vi "indexed_analog.vi"() -> ()   [LabVIEW 2018]
panel:
  in  "Index":u16
  in  "Analog":fxp<+/-,24,5>
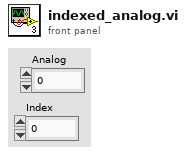
[diagram p1: front panel]
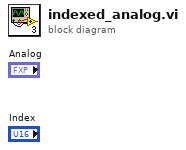
[diagram p0: block diagram]
diagram:
